vi "Teleop.vi"(10 "Match Info":T1={"Autonomous Elapsed Seconds"=0.0, "TeleOp Elapsed Seconds"=0.0, "Disabled Elapsed Seconds"=0.0, "Visited Autonomous"=FALSE, "Visited TeleOp"=FALSE, "Visited Disabled"=FALSE, "Autonomous Settings"={"Autonomous Style"=enum."Independent", "VI Refnum"=refnum}}, 11 "Call Context":T2) -> ()   [LabVIEW 2019]
doc: "This VI is called for each enabled TeleOp packet received from the DS. It is typically used to read from joysticks and other inputs and update I/O or setpoints for timed control loops. It should complete and return within 20 milliseconds or risk missing DS packets."
uses:
  <vilib>/Rock Robotics/WPI/DriverStation/WPI_DriverStationDerivedRobotMode.ctl
  <vilib>/Rock Robotics/WPI/DriverStation/WPI_DriverStationMatch Info.ctl
  <vilib>/Rock Robotics/WPI/Utilities/WPI_GetSetVariantRefNum.vi
  <vilib>/Rock Robotics/Network Tables/NT Write Boolean Array.vi
  <vilib>/Rock Robotics/Network Tables/NT Write Numeric Array.vi
  testbed-project/Support Code/initial heading.vi
  Watashi-Infinite-Recharge-San-2021/distance to target.vi
panel:
  out "distance from target":dbl
  out "Target heading":dbl
  out "Current Heading":dbl
  out "backRight":dbl
  out "backLeft":dbl
  out "frontRight":dbl
  out "frontLeft":dbl
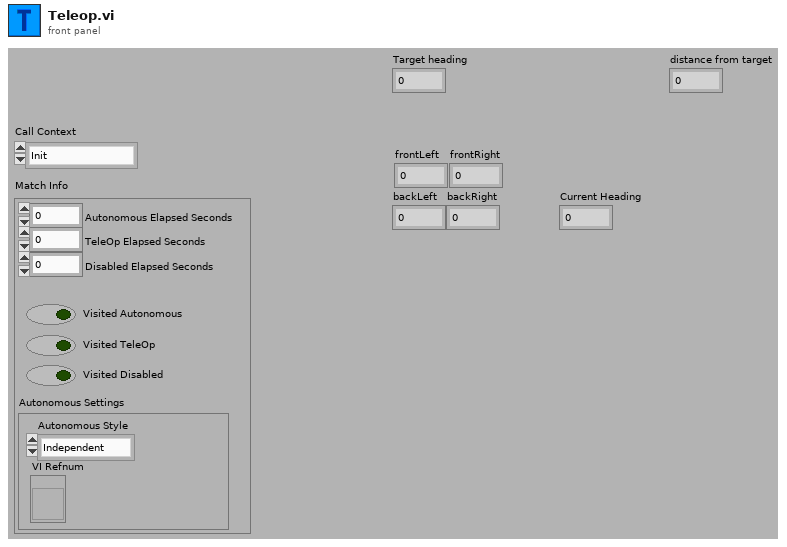
[diagram p1: front panel]
types:
  T1 = typedef "WPI_DriverStationMatch Info.ctl" = cluster{"Autonomous Elapsed Seconds":dbl, "TeleOp Elapsed Seconds":dbl, "Disabled Elapsed Seconds":dbl, "Visited Autonomous":bool, "Visited TeleOp":bool, "Visited Disabled":bool, "Autonomous Settings":cluster{"Autonomous Style":enum16{"Iterative", "Independent"}, "VI Refnum":refnum<vi>}}
  T2 = typedef "WPI_DriverStationDerivedRobotMode.ctl" = enum16{"Init", "Execute", "Stop"}
  T3 = typedef "WPI_JoystickDevRef.ctl" = cluster{"Device":T4}
  T4 = typedef "WPI_JoystickDeviceEnum.ctl" = enum16{"USB 0", "USB 1", "USB 2", "USB 3", "USB 4", "USB 5"}
  T5 = cluster{"Yaw":dbl, "Roll":dbl, "Pitch":dbl, "Heading":dbl, "Fused Heading":dbl}
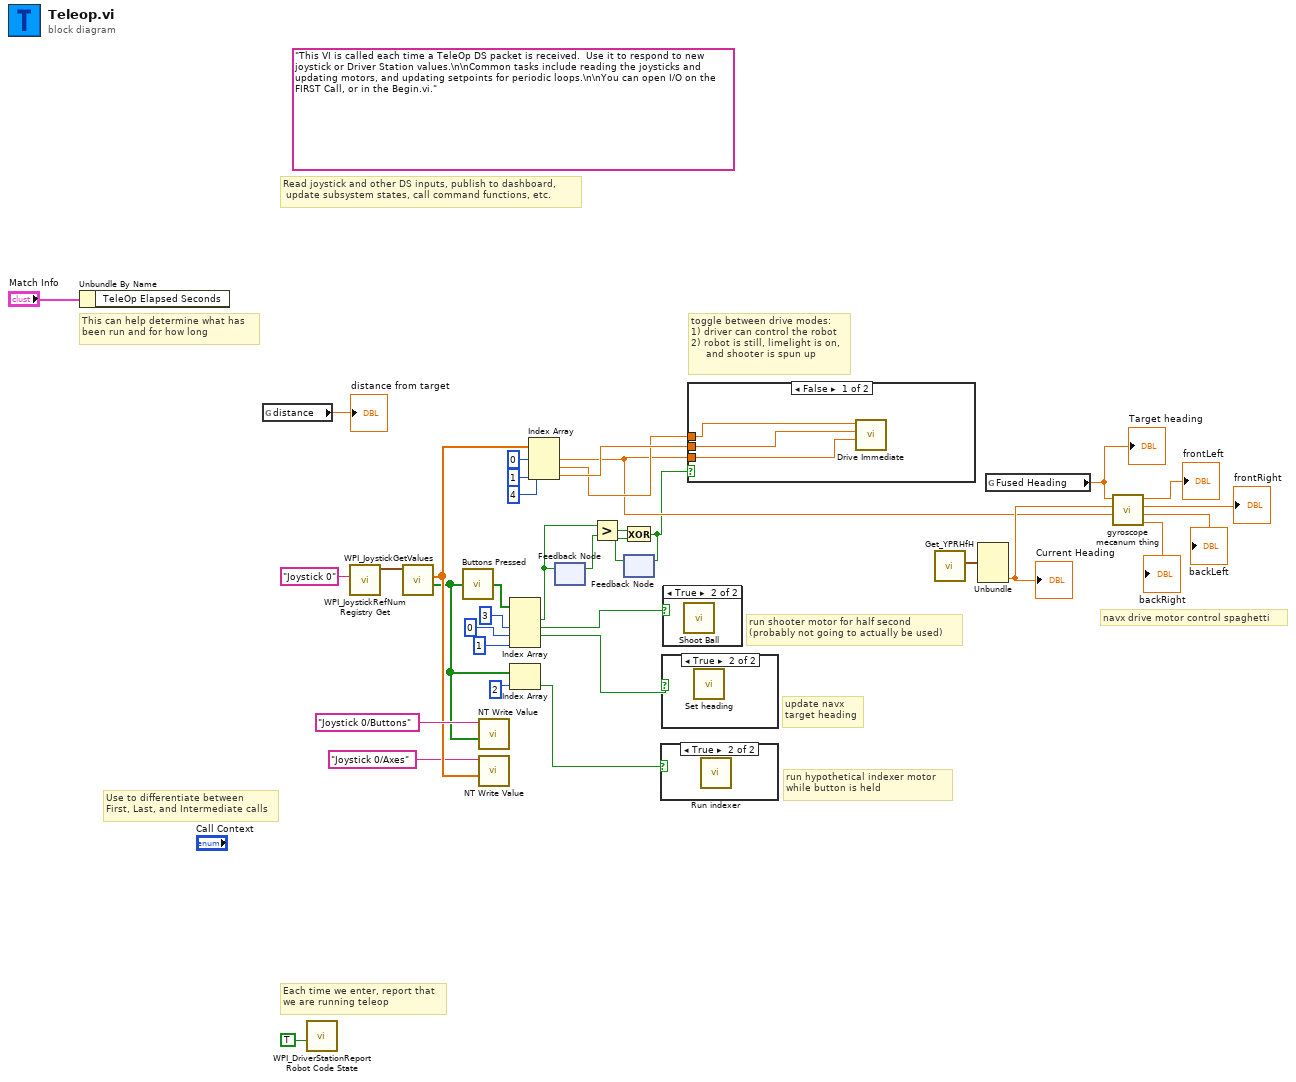
[diagram p0: block diagram]
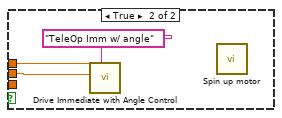
[diagram p4: hidden frame]
diagram:
  (unwired) "This VI is called each time a TeleOp DS packet is received.  Use it to respond to new joystick or Driver Station values.\n\nCommon tasks include reading the joysticks and updating motors, and updating setpoints for periodic loops.\n\nYou can open I/O on the FIRST Call, or in the Begin.vi."
  # "navx drive motor control spaghetti"
  # "toggle between drive modes:\n1) driver can control the robot\n2) robot is still, limelight is on,\n     and shooter is spun up"
  # "run hypothetical indexer motor\nwhile button is held"
  # "update navx \ntarget heading"
  # "run shooter motor for half second\n(probably not going to actually be used)"
  # "Read joystick and other DS inputs, publish to dashboard,\n update subsystem states, call command functions, etc."
  # "Each time we enter, report that\nwe are running teleop"
  # "Use to differentiate between\nFirst, Last, and Intermediate calls"
  # "This can help determine what has\nbeen run and for how long"
  n1 = Unbundle By Name("Match Info") -> ()  [unwired: 1 out]
  n2 = global read "distance to target.vi" "distance"() -> (→"distance from target":dbl)
  n3 = call <vilib>:"WPI_DriverStationReport Robot Code State.vi"("TeleOp"=TRUE ("Autonomous")) -> ()  [unwired: 10 in, 1 out]
  n4 = call <vilib>:"WPI_JoystickRefNum Registry Get.vi"("refnum name"="Joystick 0") -> ("JoystickDevRef"=w32:T3)  [unwired: 1 in, 9 out]
  n5 = call <vilib>:"WPI_JoystickGetValues.vi"("JoystickDevRef"=w32) -> ("Buttons"=w9:bool[], "Axes"=w29:dbl[])  [unwired: 6 in, 3 out]
  n6 = call "Buttons Pressed.vi"("Button Values"=w9) -> ("Button Presses"=w31:bool[])
  n7 = call-poly <vilib>:"NT Write Value.vi"("Boolean Array"=w9, "Name"="Joystick 0/Buttons") -> ()  [unwired: 9 in, 1 out]
  n8 = call-poly <vilib>:"NT Write Value.vi"("Numeric Array"=w29, "Name"="Joystick 0/Axes") -> ()  [unwired: 9 in, 1 out]
  n9 = Index Array(array=w31, index #1=1 ("index"), index #2=3 ("index"), index #3=0 ("index")) -> (element #1=w4:bool, element #2=w10:bool, element #3=w20:bool)  [unwired: 1 in, 1 out]
  n10 = Index Array(array=w9, index=2) -> (element=w7:bool)
  n11 = Index Array(array=w29, index #1=0 ("index"), index #2=1 ("index"), index #3=4 ("index")) -> (element #1=w16:dbl, element #2=w17:dbl, element #3=w18:dbl)
  n12 = feedback-in #1(w4) -> ()
  n13 = feedback #1() -> (w14:bool)  [unwired: 1 in]
  n14 = Greater?(x=w4, y=w14) -> (0:w13:bool)
  n15 = feedback #2() -> (w12:bool)  [unwired: 1 in]
  n16 = Exclusive Or(1:w12, 2:w13) -> (0:w11:bool)
  n17 = feedback-in #2(w11) -> ()
  n18 = case shown="True" w7 {
    frame False {
    }
    frame True {
      n19 = call "Run indexer.vi"() -> ()  [unwired: 11 in, 1 out]
    }
  }
  n20 = case shown="True" w20 {
    frame False {
    }
    frame True {
      n21 = call "Set heading.vi"() -> ()  [unwired: 11 in, 1 out]
    }
  }
  n22 = case shown="True" w10 {
    frame False {
    }
    frame True {
      n23 = call "Shoot Ball.vi"() -> ()  [unwired: 11 in, 1 out]
    }
  }
  n24 = case shown="False" w11 {
    tunnel: w18 -> [w37 w40]
    tunnel: w17 -> [w38 w41]
    tunnel: w16 -> [w36 _]
    frame False {
      n25 = call "Drive Immediate.vi"("Right joystick x"=w36, "Left joystick y"=w37, "Left joystick x"=w38) -> ()  [unwired: 8 in, 1 out]
    }
    frame True {
      n26 = call "Drive Immediate with Angle Control.vi"("Description"="TeleOp Imm w/ angle", "Right Setpoint"=w40, "Left Setpoint"=w41) -> ()  [unwired: 8 in, 1 out]
      n27 = call "Spin up motor.vi"() -> ()  [unwired: 11 in, 1 out]
    }
  }
  n28 = call <vilib>:"Get_YPRHfH.vi"() -> ("YRPHfH"=w26:T5)  [unwired: 11 in]
  n29 = Unbundle(w26) -> ("Fused Heading"=w25:dbl)  [unwired: 4 out]
  "Current Heading" <- w25
  n30 = global read "initial heading.vi" "Fused Heading"() -> (w19:dbl)
  "Target heading" <- w19
  n31 = call "gyroscope mecanum thing.vi"("Direction"=w16, "gyroscope position"=w25, "Target Position"=w19) -> ("backRight"=→"backRight":dbl, "backLeft"=→"backLeft":dbl, "frontRight"=→"frontRight":dbl, "frontLeft"=→"frontLeft":dbl)  [unwired: 5 in]
